vi "Set Bitpacked Channels.vi"(8 "error in (no error)":errorcluster, 10 "Item Ref in":T1 format="%.0x", 11 "Number of Channels":u8) -> (0 "error out":errorcluster)   [LabVIEW 2020, in "FPGA Addon System Explorer.lvlib"]
uses:
  FPGA Addon System Explorer.lvlib
  <vilib>/NI VeriStand/Custom Device API/Custom Device Item Ref.ctl
  Addon Shared/Types/FG Action.ctl
  <vilib>/NI VeriStand/Custom Device API/Custom Device Channel.ctl
  <vilib>/NI VeriStand/Custom Device API/Custom Device Channel Type.ctl
  Addon Shared/SubVIs/Constants.vi
  <vilib>/NI VeriStand/Custom Device Tools/Custom Device Utility Library/NI VeriStand - Search for All Items by GUID.vi
  <vilib>/NI VeriStand/Custom Device API/NI VeriStand - Get Item Property.vi
  <vilib>/NI VeriStand/Custom Device API/Get Item Property (U32).vi
  <vilib>/NI VeriStand/Custom Device API/NI VeriStand - Set Item Property.vi
  <vilib>/NI VeriStand/Custom Device API/Set Item Property (U32).vi
  Addon Shared/FPGA Addon Shared.lvlib
  <vilib>/NI VeriStand/Custom Device API/Custom Device API.lvlib
  <vilib>/NI VeriStand/Custom Device Tools/Custom Device Utility Library/Custom Device Utility Library.lvlib
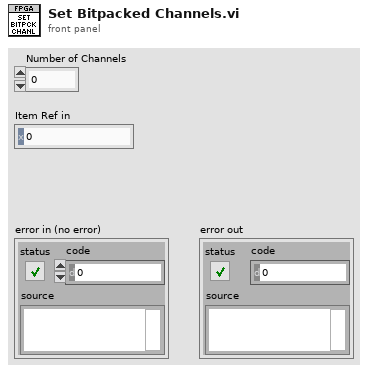
[diagram p1: front panel]
types:
  T1 = typedef "Custom Device API.lvlib/Custom Device Item Ref.ctl" = u64
  T2 = typedef "FPGA Addon Shared.lvlib/FG Action.ctl" = enum8{"GET", "SET"}
  T3 = typedef "Custom Device API.lvlib/Custom Device Item Info.ctl" = cluster{"Name":string, "Is Channel":bool, "GUID":string, "Is Waveform":bool}
  T4 = typedef "Custom Device API.lvlib/Custom Device Channel.ctl" = cluster{"Type":T5, "Units":string, "Default Value":dbl, "Faultable":bool, "Scalable":bool}
  T5 = typedef "Custom Device API.lvlib/Custom Device Channel Type.ctl" = enum16{"Input", "Output"}
  T6 = typedef "FPGA Addon Shared.lvlib/Scalar Settings.ctl" = cluster{"Number of Channels":u8}
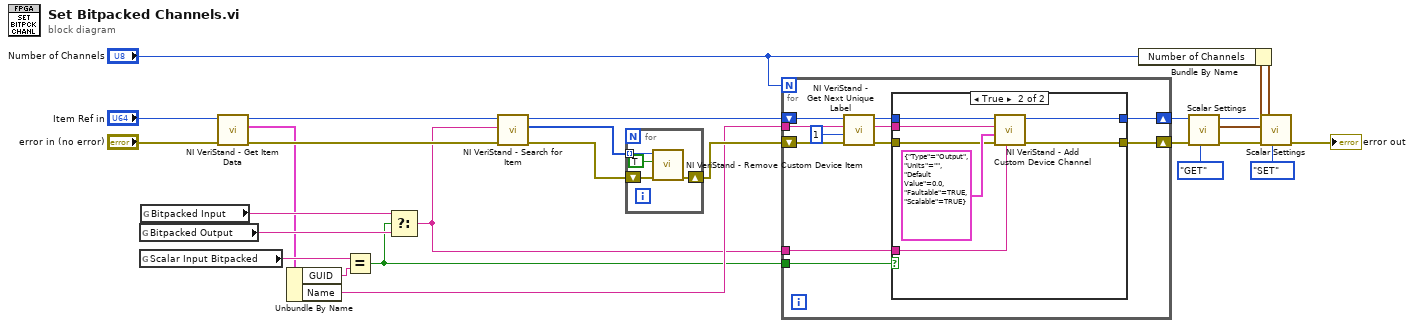
[diagram p0: block diagram]
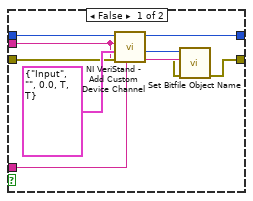
[diagram p2: hidden frame]
diagram:
  n1 = global read "Constants.vi" "Bitpacked Output"() -> (w13:string)
  n2 = global read "Constants.vi" "Scalar Input Bitpacked"() -> (w14:string)
  n3 = global read "Constants.vi" "Bitpacked Input"() -> (w12:string)
  n4 = call <vilib>:"NI VeriStand - Get Item Data.vi"("error in (no error)"="error in (no error)", "Item Ref in"="Item Ref in") -> ("error out"=w9:errorcluster, "Item Info"=w3:T3, "Item Ref out"=w4:T1)  [unwired: 7 out]
  n5 = Unbundle By Name(w3) -> ("GUID"=w11:string, "Name"=w5:string)
  n6 = Equal?(x=w14, y=w11) -> (x = y?=w2:bool)
  n7 = Select(t=w12, s=w2, f=w13) -> (s? t:f=w1:string)
  n8 = call-poly <vilib>:"NI VeriStand - Search for Item.vi"("error in"=w9, "Item GUID"=w1, "Section Ref in"=w4) -> ("error out"=w25:errorcluster, "Item Refs"=w26:T1[], "Section Ref out"=w7:T1)  [unwired: 5 in, 1 out]
  n9 = for {
    shift-right: [w29] -> w6
    shift-left: w25 -> [w30]
    tunnel: w26 -> [w27] mode=indexing
    n10 = call <vilib>:"NI VeriStand - Remove Custom Device Item.vi"("error in (no error)"=w30, "Force Delete (F)"=TRUE, "Item Ref in"=w27) -> ("error out"=w29:errorcluster)  [unwired: 7 in, 1 out]
  }
  n11 = for {
    N: "Number of Channels" -> [_]
    tunnel: w5 -> [w35]
    shift-right: [w41] -> w16
    shift-left: w6 -> [w37]
    shift-right: [w33] -> w17
    shift-left: w7 -> [w36]
    tunnel: w1 -> [w32]
    tunnel: w2 -> [w31]
    n12 = call <vilib>:"NI VeriStand - Get Next Unique Label.vi"("error in (no error)"=w37, "Start Value (1)"=1, "Label"=w35, "Parent Ref in"=w36) -> ("error out"=w40:errorcluster, "Label out"=w38:string, "Parent Ref dup"=w39:T1)  [unwired: 4 in, 1 out]
    n13 = case shown="True" w31 {
      tunnel: [w42 w53] -> w41
      tunnel: w40 -> [w48 w54]
      tunnel: w39 -> [w49 w56]
      tunnel: w38 -> [w44 w55]
      tunnel: [w47 w52] -> w33
      tunnel: w32 -> [w46 w51]
      frame False {
        n14 = call <vilib>:"NI VeriStand - Add Custom Device Channel.vi"("GUID (Default Channel)"=w46, "error in (no error)"=w48, "Channel"=T4 {"Type"=enum."Input", "Units"="", "Default Value"=0.0, "Faultable"=TRUE, "Scalable"=TRUE}, "Channel Name"=w44, "Parent Ref in"=w49) -> ("error out"=w43:errorcluster, "Channel Ref"=w45:T1, "Parent Ref out"=w47:T1)  [unwired: 3 in, 1 out]
        n15 = call "Set Bitfile Object Name.vi"("error in (no error)"=w43, "Name"=w44, "Channel Ref"=w45) -> ("error out"=w42:errorcluster)  [unwired: 8 in]
      }
      frame True {
        n16 = call <vilib>:"NI VeriStand - Add Custom Device Channel.vi"("GUID (Default Channel)"=w51, "error in (no error)"=w54, "Channel"=T4 {"Type"=enum."Output", "Units"="", "Default Value"=0.0, "Faultable"=TRUE, "Scalable"=TRUE}, "Channel Name"=w55, "Parent Ref in"=w56) -> ("error out"=w53:errorcluster, "Parent Ref out"=w52:T1)  [unwired: 3 in, 2 out]
      }
    }
  }
  n17 = call "Scalar Settings.vi"("Action"=FG_Action."GET", "error in (no error)"=w16, "Item Ref"=w17) -> ("error out"=w20:errorcluster, "Scalar Settings"=w22:T6, "Item Ref out"=w19:T1)  [unwired: 6 in]
  n18 = Bundle By Name(cluster=w22, "Number of Channels"="Number of Channels") -> (w23:T6)
  n19 = call "Scalar Settings.vi"("Action"=FG_Action."SET", "error in (no error)"=w20, "Scalar Settings"=w23, "Item Ref"=w19) -> ("error out"=→"error out":errorcluster)  [unwired: 5 in, 2 out]
